vi "Get API Key.vi"(8 "Error In":errorcluster, 11 "Open Weather Session In":refnum<class "Open Weather Session.lvclass">) -> (0 "Error Out":errorcluster, 2 "API Key":string, 3 "Open Weather Session Out":refnum<class "Open Weather Session.lvclass">)   [LabVIEW 2019, in "Open Weather Session.lvclass"]
uses:
  Open Weather Session.lvclass
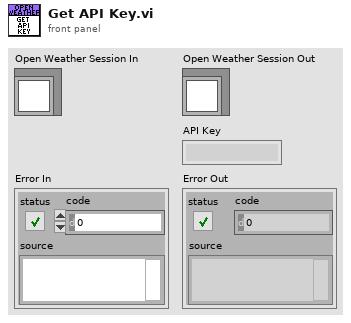
[diagram p1: front panel]
types:
  T1 = typedef "Open Weather Session.lvclass/Data.ctl" = cluster{"API Key":string, "REST Client":refnum<class "REST Client.lvclass">}
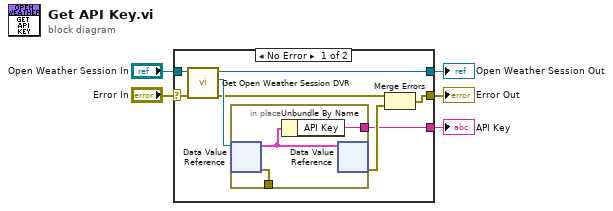
[diagram p0: block diagram]
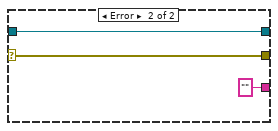
[diagram p2: hidden frame]
diagram:
  n1 = case shown="No Error" "Error In" {
    selector: "Error In" -> [w9 w18]
    tunnel: [w11 w18] -> w2
    tunnel: [w8 w19] -> w4
    tunnel: "Open Weather Session In" -> [w10 w19]
    tunnel: [w12 "" ("API Key")] -> w1
    frame No Error {
      n2 = call "Get Open Weather Session DVR.vi"("Error In"=w9, "Open Weather Session In"=w10) -> ("Error Out"=w6:errorcluster, "DVR"=w7:refnum<data-value>, "Open Weather Session Out"=w8:refnum<class "Open Weather Session.lvclass">)  [unwired: 7 in]
      n3 = in-place {
        in-place-border: [w14] -> w12
        in-place-border: [w16] -> _
        n4 = in-place-dvr #1(w7) -> (w15:T1, w16:errorcluster)
        n5 = Unbundle By Name(w15) -> ("API Key"=w14:string)
        n6 = in-place-dvr #1(w15) -> (w13:errorcluster)  [unwired: 1 out]
      }
      n7 = Merge Errors(w6, w13) -> (w11:errorcluster)
    }
    frame Error {
    }
  }
  "Open Weather Session Out" <- w4
  "Error Out" <- w2
  "API Key" <- w1
